vi "addArrayElement.vi"(8 "error in (no error)":errorcluster, 9 "arraySize":u16, 10 "arrayRef":refnum<vi>, 11 "Primitive in":refnum<class "Primitive.lvclass">) -> (0 "error out":errorcluster, 2 "arrayRef 2":refnum<vi>, 3 "Primitive out":refnum<class "Primitive.lvclass">)   [LabVIEW 2016, in "Primitive.lvclass"]
uses:
  Primitive.lvclass
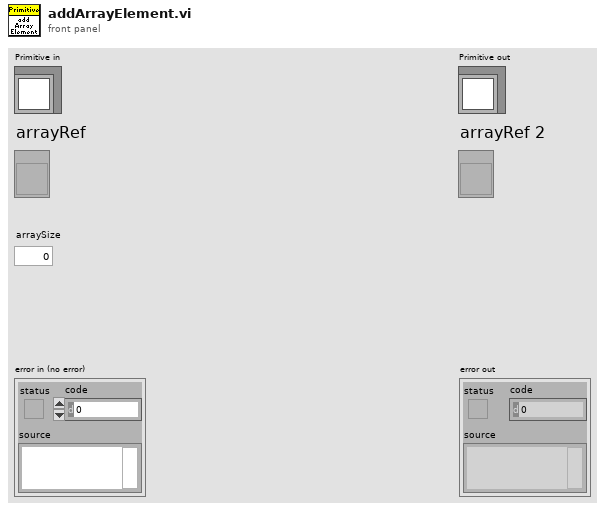
[diagram p1: front panel]
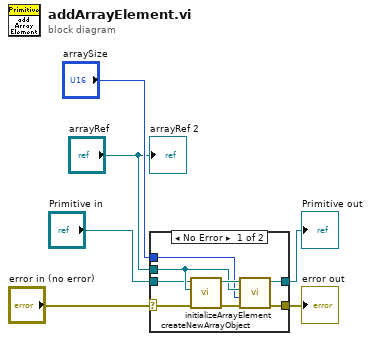
[diagram p0: block diagram]
diagram:
  n1 = case shown="No Error" "error in (no error)" {
    selector: "error in (no error)" -> [w10 w16]
    tunnel: [w9 w16] -> w5
    tunnel: [w7 w15] -> w3
    tunnel: "Primitive in" -> [w8 w15]
    tunnel: "arrayRef" -> [w12 _]
    tunnel: "arraySize" -> [w11 _]
    frame No Error {
      n2 = call-dynamic "createNewArrayObject.vi"("error in (no error)"=w10, "arrayRef"=w12, "Primitive in"=w8) -> ("error out"=w13:errorcluster, "Primitive out"=w14:refnum<class "Primitive.lvclass">)  [unwired: 7 in]
      n3 = call-dynamic "initializeArrayElement.vi"("error in (no error)"=w13, "arraySize"=w11, "arrayRef"=w12, "Primitive in"=w14) -> ("error out"=w9:errorcluster, "Primitive out"=w7:refnum<class "Primitive.lvclass">)  [unwired: 6 in]
    }
    frame Error {
    }
  }
  "error out" <- w5
  "Primitive out" <- w3
  "arrayRef 2" <- "arrayRef"
